vi "PSETEX.vi"(0 "TCP session out":refnum<k5>, 1 "Key":string, 5 "Milliseconds":string, 7 "Value":string, 11 "error in":errorcluster) -> (4 "TCP session out":refnum<k5>, 6 "Data":T1, 15 "error out":errorcluster)   [LabVIEW 2023]
uses:
  SubVIs/Controls/redis-data.ctl
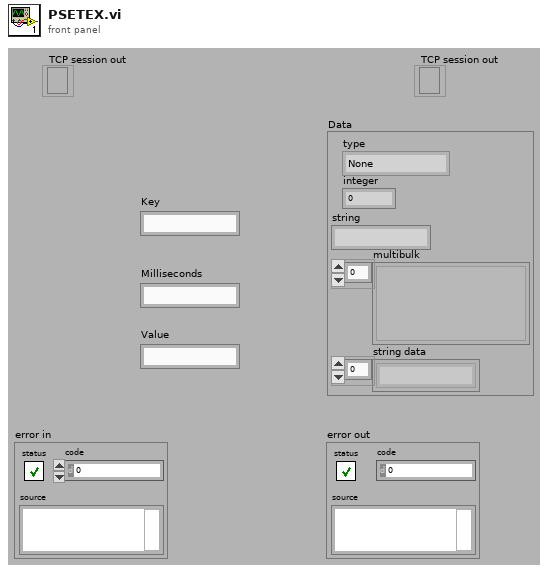
[diagram p1: front panel]
types:
  T1 = typedef "redis-data.ctl" = cluster{"type":enum16{"None", "Error", "Status", "Nil", "Integer", "String", "Multibulk"}, "integer":i64, "string":string, "multibulk":variant[], "string data":string[]}
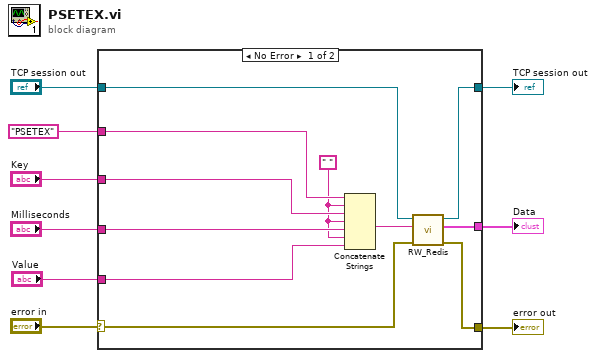
[diagram p0: block diagram]
diagram:
  n1 = case shown="No Error" "error in" {
    selector: "error in" -> [w19 w22]
    tunnel: "PSETEX" -> [w16 _]
    tunnel: "TCP session out" -> [w13 w21]
    tunnel: [w18 w22] -> w7
    tunnel: [w17 _] -> w3
    tunnel: "Key" -> [w15 _]
    tunnel: "Milliseconds" -> [w14 _]
    tunnel: [w10 w21] -> w2
    tunnel: "Value" -> [w11 _]
    frame No Error {
      w12 = " "
      n2 = Concatenate Strings(w16, w12, w15, w12, w14, w12, w11) -> (w20:string)
      n3 = call "RW_Redis.vi"("error in"=w19, "command"=w20, "TCP session in"=w13) -> ("error out"=w18:errorcluster, "Data"=w17:T1, "TCP session out"=w10:refnum<k5>)  [unwired: 6 in]
    }
    frame Error {
    }
  }
  "error out" <- w7
  "TCP session out" <- w2
  "Data" <- w3
